vi "_hla_messaging_coordinator.vi"(1 "actions":T2, 2 "fom_path (in)":path, 3 "params":T1, 5 "error in (no error)":errorcluster) -> (16 "controlled_event_ref (out)":refnum<user-event>, 19 "error out":errorcluster)   [LabVIEW 2016]
doc: "The HLA Messaging Communicator is the primary utility for controlling, both directly and indirectly, HLA message transactions to and from the Federation to which this Federate is a part of. Recall that, for a LabVIEW based federate to actively participate in a Federation (and in part be managed by a Federation Manager), it must subscribe to the same set of rules as any other Federate in the simulation. Because LabVIEW in of itself is abstract from the native Java implementation of Federates, there exists a Java component (the HLA Adapter) that, when combined with a custom LabVIEW application, forms what is considered the complete LabVIEW federate. The two communicate with one another over dedicated sockets for receiving messages (where the adapter is the server) and sending messages (where the LabVIEW code acts as the server).\n\nAs of this writing, there are currently (3) actions available to the Communicator:\n\n<B>activate</B> - call this action to initialize the communicator by establlishing proper TCP connections with the Java component to this custom federate. There are two required inputs when this action is invoked: <B>params</B> and <B>fom_path</B>. More on these below.\n<B>terminate</B> - call this action to properly close out communications and any open TCP connections\n<B>get_event_ref</B> - call this action to pull the custom events reference to assist in the management of event-triggering messages such as advancing logical time (do-step), handling requests to end the simulation (sim-end) and simply aborting (abort).\n\n<B>Required Inputs for the \"activate\" action:</B>\nBefore executing the <B>activate</B> action, certain inputs are required as inputs. The params cluster contains three values that MUST be included:\n\n<B>hla_adapter_ip</B> - The IP address of the host machine running the Java based adapter component to this federate. \n<B>hla_adapter_port</B> - The specicied port to open a TCP socket for receiving messages from the Java based adapter component to this federate\n<B>listener_port</B> the local port (where this LabVIEW code will be running) to which the Java based adapter component will establish a connection for receiving messages from custom written LabVIEW code\n\nLastly, the file path to the FOM file. This is the same FOM file used to pre-build the suite of federate library code specifially used for receiving/sending interations and objects."
uses:
  support/controls/hla_messaging_coordinator_actions.ctl
  support/controls/messaging_processor_params.ctl
  support/controls/user_event_item.ctl
  support/controls/user_events.ctl
  support/controls/messaging_processor_handler_actions.ctl
  support/controls/queue_assistant_actions.ctl
  support/controls/event_assistant_actions.ctl
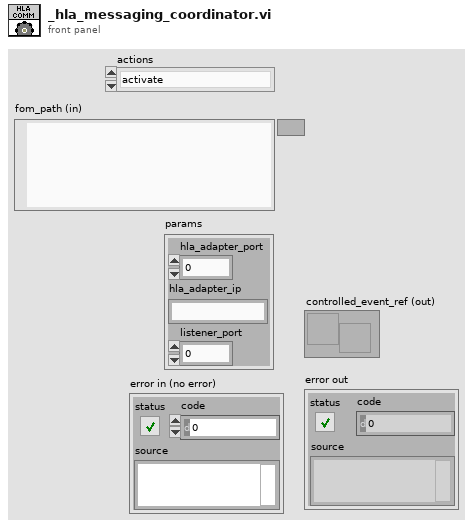
[diagram p1: front panel]
types:
  T1 = typedef "messaging_processor_params.ctl" = cluster{"hla_adapter_port":u16, "hla_adapter_ip":string, "listener_port":u16}
  T2 = typedef "hla_messaging_coordinator_actions.ctl" = enum16{"activate", "get_event_ref", "terminate"}
  T3 = typedef "event_assistant_actions.ctl" = enum16{"--- unused ---", "destroy", "fire", "get_ref", "init"}
  T4 = typedef "queue_assistant_actions.ctl" = enum16{"--- unused ---", "bulk_enq_ahead", "bulk_enq_behind", "destroy", "empty?", "enq_ahead", "enq_behind", "flush", "get_queues", "init"}
  T5 = typedef "messaging_processor_handler_actions.ctl" = enum16{"------ unused ------", "close", "init", "launch", "run"}
  T6 = typedef "raw_object_interaction_descriptor.ctl" = cluster{"classpath (id)":string, "shortname":string, "param_names":string[], "param_dtypes":string[]}
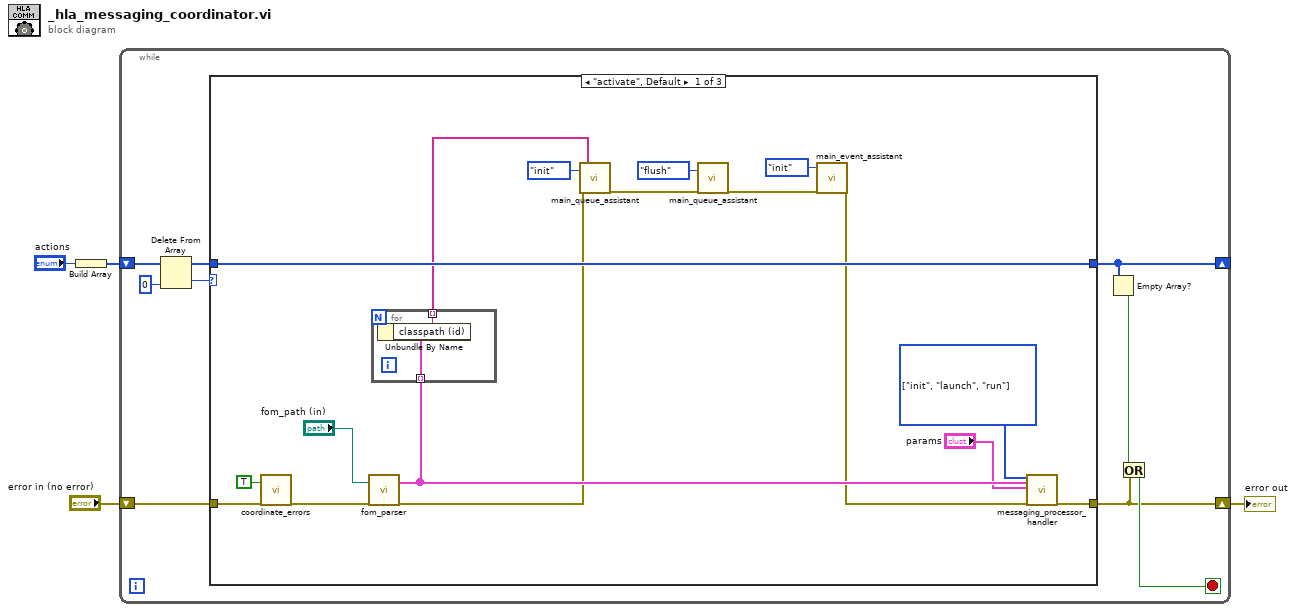
[diagram p0: block diagram]
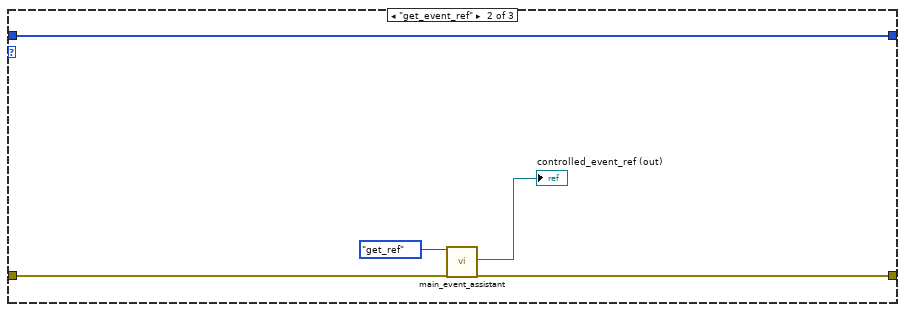
[diagram p2: hidden frame]
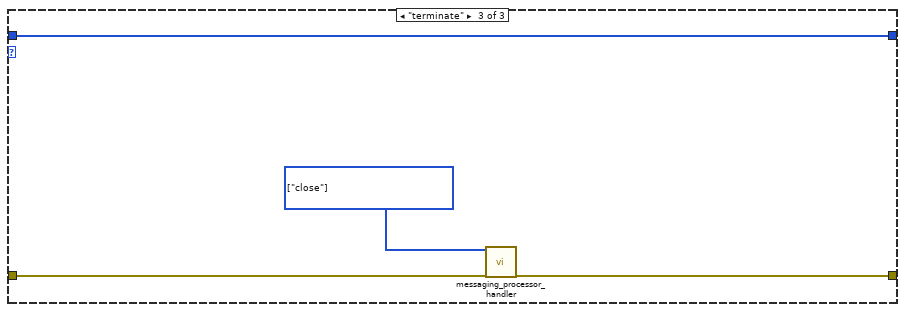
[diagram p3: hidden frame]
diagram:
  n1 = Build Array("actions") -> (w3:T2[])
  n2 = while {
    shift-right: [w9] -> _
    shift-left: w3 -> [w13]
    shift-right: [w5] -> w1
    shift-left: "error in (no error)" -> [w8]
    stop <- w6 stop-if-true
    n3 = Delete From Array(array=w13, index=0) -> (deleted portion=w11:T2, array with subset deleted=w10:T2[])  [unwired: 1 in]
    n4 = case shown="\"activate\", Default" w11 {
      tunnel: w10 -> [w27 w36 w40]
      tunnel: [w27 w36 w40] -> w9
      tunnel: w8 -> [w30 w35 w39]
      tunnel: [w28 w34 w41] -> w5
      frame "activate", Default {
        w24 = T5[] [enum."init", enum."launch", enum."run"] items=["------ unused ------", "close", "init", "launch", "run"] ("actions")
        n5 = call "coordinate_errors.vi"("reset"=TRUE, "error in (no error)"=w30) -> ("error"=w26:errorcluster)  [unwired: 16 in, 1 out]
        n6 = call "fom_parser.vi"("fom_path (in)"="fom_path (in)", "error in (no error)"=w26) -> ("interaction_descriptors (out)"=w20:T6[], "error out"=w18:errorcluster)  [unwired: 16 in]
        n7 = for {
          tunnel: w20 -> [w32] mode=indexing
          tunnel: [w31] -> w19 mode=indexing
          n8 = Unbundle By Name(w32) -> ("classpath (id)"=w31:string)
        }
        n9 = call "main_queue_assistant.vi"("action (enq_behind = def)"=queue_assistant_actions."init" ("queue_action (enq_behind = def)"), "error in (no error)"=w18, "classpaths_for_queue_identification (ids)"=w19) -> ("error out"=w21:errorcluster)  [unwired: 14 in, 2 out]
        n10 = call "main_queue_assistant.vi"("action (enq_behind = def)"=queue_assistant_actions."flush" ("queue_action (enq_behind = def)"), "error in (no error)"=w21) -> ("error out"=w17:errorcluster)  [unwired: 15 in, 2 out]
        n11 = call "main_event_assistant.vi"("event_action (enq_behind = def)"=event_assistant_actions."init", "error in (no error)"=w17) -> ("error out"=w16:errorcluster)  [unwired: 16 in, 1 out]
        n12 = call "messaging_processor_handler.vi"("actions"=w24, "interaction_descriptors (in)"=w20, "params"="params", "error in (no error)"=w16) -> ("error out"=w28:errorcluster)  [unwired: 15 in]
      }
      frame "get_event_ref" {
        n13 = call "main_event_assistant.vi"("event_action (enq_behind = def)"=event_assistant_actions."get_ref", "error in (no error)"=w35) -> ("controlled event"=→"controlled_event_ref (out)":refnum<user-event>, "error out"=w34:errorcluster)  [unwired: 16 in]
      }
      frame "terminate" {
        w38 = T5[] [enum."close"] items=["------ unused ------", "close", "init", "launch", "run"] ("actions")
        n14 = call "messaging_processor_handler.vi"("actions"=w38, "error in (no error)"=w39) -> ("error out"=w41:errorcluster)  [unwired: 17 in]
      }
    }
    n15 = Empty Array?(array=w9) -> (empty?=w7:bool)
    n16 = Or(x=w7, y=w5) -> (x .or. y?=w6:bool)
  }
  "error out" <- w1
